vi "Get Plugin Relative Path.vi"(11 "File Path":path=path "C:/Users/Public/Documents/CIF/plugins/files/loggers/mycode") -> (3 "Relative Path":string[](array[string]))   [LabVIEW 2021, in "CIFPluginLoader.lvclass"]
uses:
  CIFPluginLoader.lvclass
  <vilib>/CIF Foundation/CIF Core/CIFUtilities/CIFConfigurationFile/typedef/Location Type.ctl
  <vilib>/CIF Foundation/CIF Core/CIFUtilities/CIFConfigurationFile/CIF Configuration File Location.vi
  <vilib>/CIF Foundation/CIF Core/CIFUtilities/CIFConfigurationFile/CIF Configuration File.lvlib
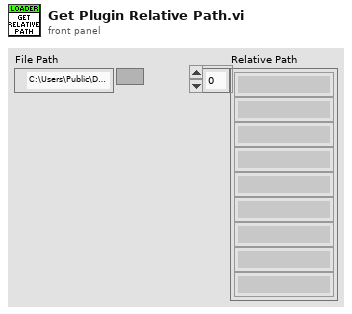
[diagram p1: front panel]
types:
  T1 = typedef "CIF Configuration File.lvlib/Location Type.ctl" = enum16{"Config File", "Manager", "Protos", "Plugins", "UI Plugins", "Logs", "Orchestrations", "Loaders"}
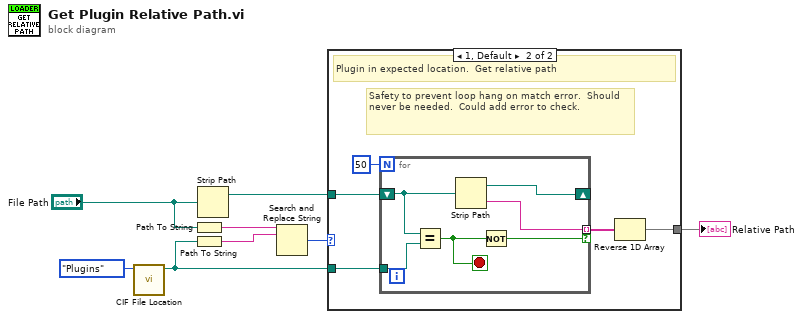
[diagram p0: block diagram]
diagram:
  n1 = call <vilib>:"CIF File Location.vi"("LocationType"=Location_Type."Plugins") -> ("Location"=w4:path)  [unwired: 10 in]
  n2 = Path To String(path="File Path") -> (string=w3:string)
  n3 = Path To String(path=w4) -> (string=w2:string)
  n4 = Strip Path(path="File Path") -> (stripped path=w7:path)  [unwired: 1 out]
  n5 = Search and Replace String(input string=w3, search string=w2) -> (number of replacements=w1:i32)  [unwired: 6 in, 3 out]
  n6 = case shown="1, Default" w1 {
    tunnel: w7 -> [_ w13]
    tunnel: [_ w11] -> w6
    tunnel: w4 -> [_ w10]
    frame 0 {
      # "Plugin is not in expected path.  Should never happen, could add error"
    }
    frame 1, Default {
      # "Safety to prevent loop hang on match error.  Should never be needed.  Could add error to check."
      # "Plugin in expected location.  Get relative path"
      n7 = for {
        N: 50 -> [_]
        tunnel: w10 -> [w19]
        shift-right: [w17] -> _
        shift-left: w13 -> [w18]
        tunnel: [w16] -> w12 mode=indexing if=w14
        stop <- w15 stop-if-true
        n8 = Equal?(x=w18, y=w19) -> (x = y?=w15:bool)
        n9 = Strip Path(path=w18) -> (stripped path=w17:path, name=w16:string)
        n10 = Not(x=w15) -> (.not. x?=w14:bool)
      }
      n11 = Reverse 1D Array(array=w12) -> (reversed array=w11:string[])
    }
  }
  "Relative Path" <- w6
